vi "Read.vi"(8 "error in (no error)":errorcluster, 10 "ILC in":refnum<class "ILC.lvclass">, 11 "ILC DAC in":refnum<class "ILC DAC.lvclass">) -> (0 "error out":errorcluster, 1 "Value":u16, 2 "ILC out":refnum<class "ILC.lvclass">, 3 "ILC DAC out":refnum<class "ILC DAC.lvclass">)   [LabVIEW 2015]
uses:
  ILC DAC.lvclass
  <userlib>/Common/ILC/ILC/ILC.lvclass
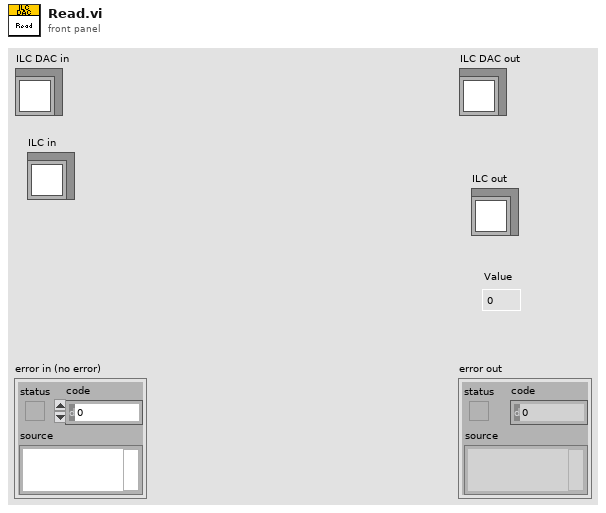
[diagram p1: front panel]
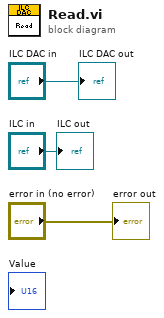
[diagram p0: block diagram]
diagram:
  "error out" <- "error in (no error)"
  "ILC DAC out" <- "ILC DAC in"
  "ILC out" <- "ILC in"
